vi "Example Simple.vi"() -> ()   [LabVIEW 2013]
uses:
  C:/tf/play/labview/Tinkerforge.dll
  Tinkerforge.dll
panel:
  in  "uid":string="abc"
  in  "port":i32=4223
  in  "host":string="localhost"
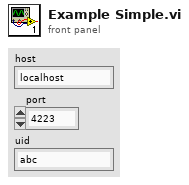
[diagram p1: front panel]
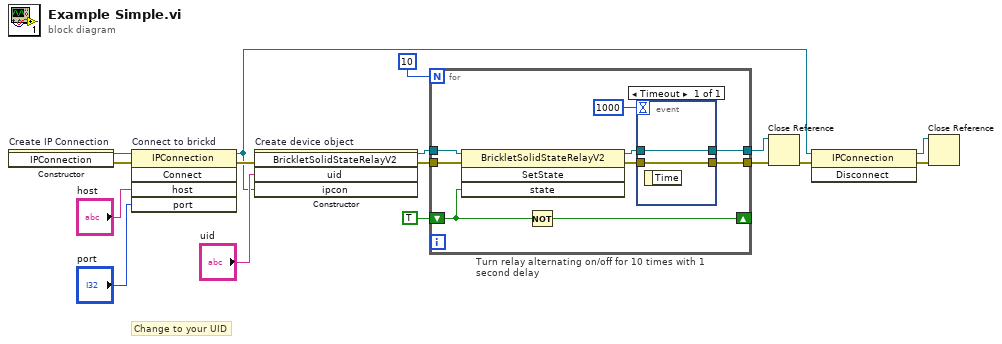
[diagram p0: block diagram]
diagram:
  # "Change to your UID"
  n1 = constructor on="Create IP Connection" class="IPConnection"() -> (reference out=w16:refnum<k24>, error out=w7:errorcluster)  [unwired: 3 in, 1 out]
  n2 = invoke on="Connect to brickd" class="IPConnection" method="Connect"(reference=w16, error in=w7, "host"="host", "port"="port") -> (reference out=w9:refnum<k24>, error out=w12:errorcluster)  [unwired: 1 in, 3 out]
  n3 = constructor on="Create device object" class="BrickletSolidStateRelayV2"(error in=w12, "uid"="uid", "ipcon"=w9) -> (reference out=w3:refnum<k24>, error out=w4:errorcluster)  [unwired: 2 in, 3 out]
  n4 = for "Turn relay alternating on/off for 10 times with 1 second delay" {
    N: 10 -> [_]
    tunnel: w4 -> [w25]
    tunnel: w3 -> [w24]
    tunnel: [w20] -> w2
    tunnel: [w22] -> w1
    shift-right: [w17] -> _
    shift-left: TRUE -> [w18]
    n5 = invoke class="BrickletSolidStateRelayV2" method="SetState"(reference=w24, error in=w25, "state"=w18) -> (reference out=w21:refnum<k24>, error out=w19:errorcluster)  [unwired: 1 in, 2 out]
    n6 = Not(x=w18) -> (.not. x?=w17:bool)
    n7 = event shown="[0] Timeout" {
      selector: _ -> [_]
      dyn-events: _ -> [_]
      timeout: 1000 -> [_]
      tunnel: [w27] -> w22
      tunnel: w21 -> [w27]
      tunnel: [w26] -> w20
      tunnel: w19 -> [w26]
      event Timeout {
        n8 = event-data() -> ()  [unwired: 1 in, 1 out]
      }
    }
  }
  n9 = Close Reference(reference=w1, error in (no error)=w2) -> (error out=w11:errorcluster)
  n10 = invoke class="IPConnection" method="Disconnect"(reference=w9, error in=w11) -> (reference out=w8:refnum<k24>, error out=w10:errorcluster)  [unwired: 1 in, 1 out]
  n11 = Close Reference(reference=w8, error in (no error)=w10) -> ()  [unwired: 1 out]
